vi "ProbeQueue.vi"(8 "error in (no error)":errorcluster, 11 "Devices queue in":refnum<queue>) -> (0 "error out":errorcluster, 3 "Devices queue out":refnum<queue>)   [LabVIEW 2013]
uses:
  DeviceVIs/Device/Device.lvclass
panel:
  out "elements":T1(array[cluster])
  out "# pending insert":i32
  out "# pending remove":i32
  out "# elements in queue":i32
  out "queue name":string
  out "max queue size":i32
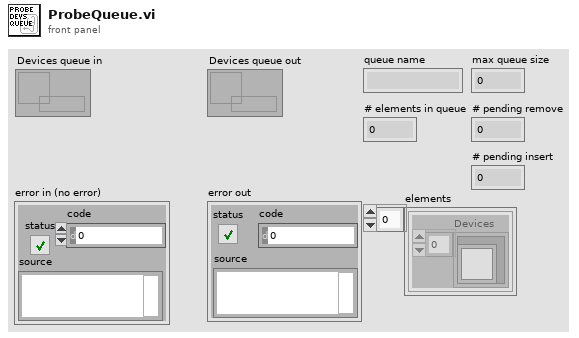
[diagram p1: front panel]
types:
  T1 = cluster{"Devices":refnum<class "Device.lvclass">[]}[]
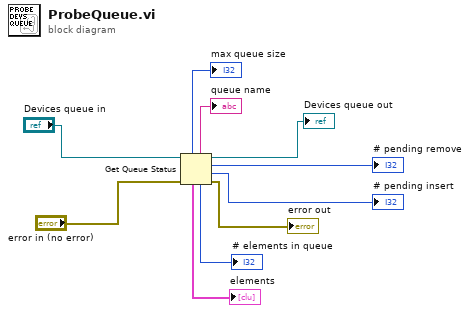
[diagram p0: block diagram]
diagram:
  n1 = Get Queue Status(queue="Devices queue in", error in (no error)="error in (no error)") -> (queue out=→"Devices queue out":refnum<queue>, queue name=→"queue name":string, max queue size=→"max queue size":i32, # pending remove=→"# pending remove":i32, # pending insert=→"# pending insert":i32, error out=→"error out":errorcluster, # elements in queue=→"# elements in queue":i32, elements=→"elements":T1)  [unwired: 1 in]
